vi "Config External Network Parameters.vi"(10 "External Network Parameters":T1) -> (2 "Parameters As Expressions":string[](array[string]))   [LabVIEW 2016, in "QPA Measurement.lvlib" / "QPA Measurement.lvclass"]
uses:
  QPA Measurement.lvclass
  Controls/External Network Parameters.ctl
  Controls/LoadPull State.ctl
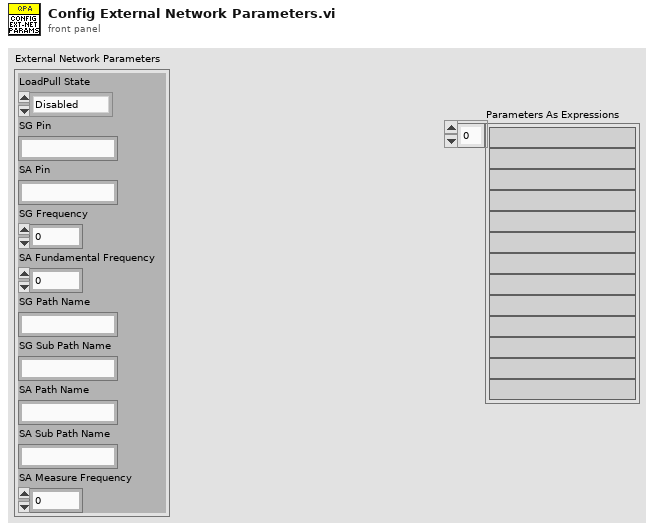
[diagram p1: front panel]
types:
  T1 = typedef "QPA Measurement.lvlib/QPA Measurement.lvclass/External Network Parameters.ctl" = cluster{"LoadPull State":T2, "SG Pin":string, "SA Pin":string, "SG Frequency":dbl, "SA Fundamental Frequency":dbl, "SG Path Name":string, "SG Sub Path Name":string, "SA Path Name":string, "SA Sub Path Name":string, "SA Measure Frequency":dbl}
  T2 = typedef "QPA Measurement.lvlib/QPA Measurement.lvclass/LoadPull State.ctl" = enum16{"Disabled", "Coupled Path", "Uncoupled Path", "Auto"}
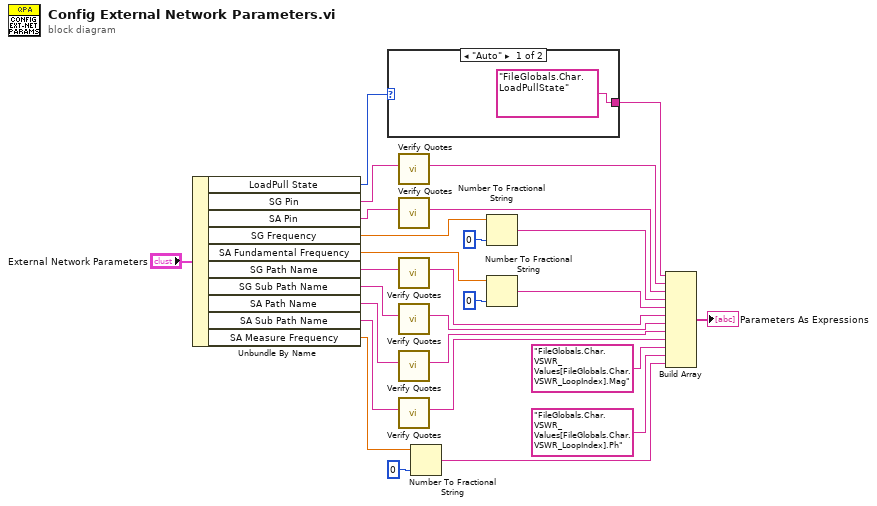
[diagram p0: block diagram]
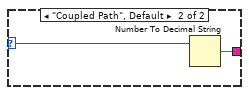
[diagram p2: hidden frame]
diagram:
  n1 = Unbundle By Name("External Network Parameters") -> ("LoadPull State"=w26:T2, "SG Pin"=w24:string, "SA Pin"=w22:string, "SG Frequency"=w21:dbl, "SA Fundamental Frequency"=w17:dbl, "SG Path Name"=w15:string, "SG Sub Path Name"=w14:string, "SA Path Name"=w13:string, "SA Sub Path Name"=w12:string, "SA Measure Frequency"=w10:dbl)
  n2 = case shown="\"Auto\"" w26 {
    selector: w26 -> [_ w30]
    tunnel: ["FileGlobals.Char.LoadPullState" w29] -> w25
    frame "Auto" {
    }
    frame "Coupled Path", Default {
      n3 = Number To Decimal String(number=w30) -> (decimal integer string=w29:string)  [unwired: 1 in]
    }
  }
  n4 = call "Verify Quotes.vi"("String In"=w24) -> ("Quote Verified String Out"=w7:string)  [unwired: 10 in]
  n5 = call "Verify Quotes.vi"("String In"=w22) -> ("Quote Verified String Out"=w6:string)  [unwired: 10 in]
  n6 = call "Verify Quotes.vi"("String In"=w15) -> ("Quote Verified String Out"=w5:string)  [unwired: 10 in]
  n7 = call "Verify Quotes.vi"("String In"=w14) -> ("Quote Verified String Out"=w4:string)  [unwired: 10 in]
  n8 = call "Verify Quotes.vi"("String In"=w13) -> ("Quote Verified String Out"=w3:string)  [unwired: 10 in]
  n9 = call "Verify Quotes.vi"("String In"=w12) -> ("Quote Verified String Out"=w2:string)  [unwired: 10 in]
  n10 = Number To Fractional String(number=w10, precision (6)=i16 0) -> (F-format string=w1:string)  [unwired: 2 in]
  n11 = Number To Fractional String(number=w21, precision (6)=i16 0) -> (F-format string=w19:string)  [unwired: 2 in]
  n12 = Number To Fractional String(number=w17, precision (6)=i16 0) -> (F-format string=w16:string)  [unwired: 2 in]
  n13 = Build Array(w25, w7, w6, w19, w16, w5, w4, w3, w2, "FileGlobals.Char.VSWR_Values[FileGlobals.Char.VSWR_LoopIndex].Mag", "FileGlobals.Char.VSWR_Values[FileGlobals.Char.VSWR_LoopIndex].Ph", w1) -> (→"Parameters As Expressions":string[])
